vi "extract plot instructions from control update.vi"(10 "OldVal":T1[](array[typedef]), 11 "Plot Control":T1[](array[typedef])) -> (1 "correctControl":T1[](array[typedef]), 3 "plotUpdate":cluster{"X":u16[], "Y":u16[], "Y2":u16[]})   [LabVIEW 2018]
uses:
  plotControl.ctl
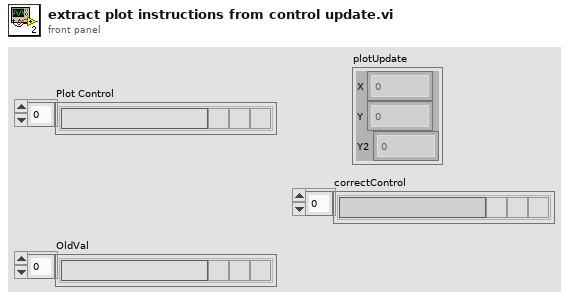
[diagram p1: front panel]
types:
  T1 = typedef "plotControl.ctl" = cluster{"channel":string, "X":bool, "Y":bool, "Y2":bool}
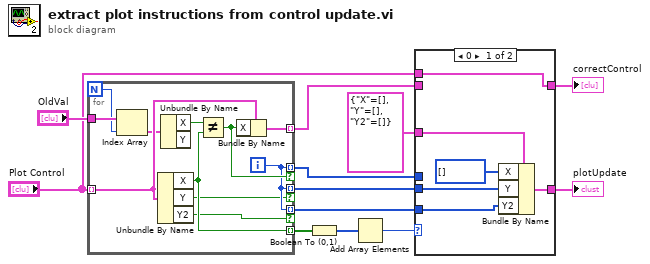
[diagram p0: block diagram]
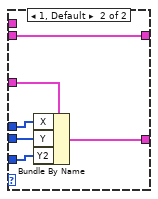
[diagram p2: hidden frame]
diagram:
  n1 = for {
    N -> [w16]
    tunnel: "OldVal" -> [w18]
    tunnel: "Plot Control" -> [w21] mode=indexing
    tunnel: [w22] -> w11 mode=indexing
    tunnel: [w15] -> w7 mode=indexing if=w14
    tunnel: [w15] -> w6 mode=indexing if=w19
    tunnel: [w20] -> w3 mode=indexing
    tunnel: [w15] -> w1 mode=indexing if=w13
    i -> [w15]
    n2 = Index Array(array=w18, index=w16) -> (element=w17:T1)
    n3 = Unbundle By Name(w21) -> ("X"=w22:bool, "Y"=w14:bool, "Y2"=w13:bool)
    n4 = Unbundle By Name(w17) -> ("X"=w23:bool)  [unwired: 1 out]
    n5 = Not Equal?(x=w23, y=w22) -> (x != y?=w19:bool)
    n6 = Bundle By Name(cluster=w21, "X"=w19) -> (w20:T1)
  }
  n7 = Boolean To (0,1)(Boolean=w11) -> (0, 1=w8:i16[])
  n8 = Add Array Elements(numeric array=w8) -> (sum=w10:i16)
  n9 = case shown="0" w10 {
    tunnel: cluster{"X":u16[], "Y":u16[], "Y2":u16[]} {"X"=[], "Y"=[], "Y2"=[]} ("plot") -> [w29 w35]
    tunnel: [w28 w34] -> w5
    tunnel: w7 -> [w26 w33]
    tunnel: w6 -> [_ w32]
    tunnel: "Plot Control" -> [w25 _]
    tunnel: [w25 w31] -> w2
    tunnel: w3 -> [_ w31]
    tunnel: w1 -> [w24 w30]
    frame 0 {
      n10 = Bundle By Name(cluster=w29, "X"=u16[] [], "Y"=w26, "Y2"=w24) -> (w28:cluster{"X":u16[], "Y":u16[], "Y2":u16[]})
    }
    frame 1, Default {
      n11 = Bundle By Name(cluster=w35, "X"=w32, "Y"=w33, "Y2"=w30) -> (w34:cluster{"X":u16[], "Y":u16[], "Y2":u16[]})
    }
  }
  "plotUpdate" <- w5
  "correctControl" <- w2
